vi "CRYControlCRY6181.vi"(0 "Command":string) -> (3 "Success?":bool, 4 "Margin":dbl, 6 "Table":string, 8 "Xdatapoints":dbl[](array[numeric]), 10 "Ydatapoints":dbl[](array[numeric]), 14 "Pass?":bool, 15 "Zdatapoints":dbl[](array[numeric]))   [LabVIEW 2013]
uses:
  CRYProject/CRYProject Editor Global.vi
  CRYMainGlobal.vi
  CRYWindow/SubVI/CRYMain Sub Window Global.vi
  CRYSystem/Task Sequence/CRYProject Run Control Global.vi
panel:
  # "run\nlot 121\nserial N1223\nexit\nopen I:\\__Test Sequence\\TSR THD.cry\ncurve Fundamental Harmonic \nnames"
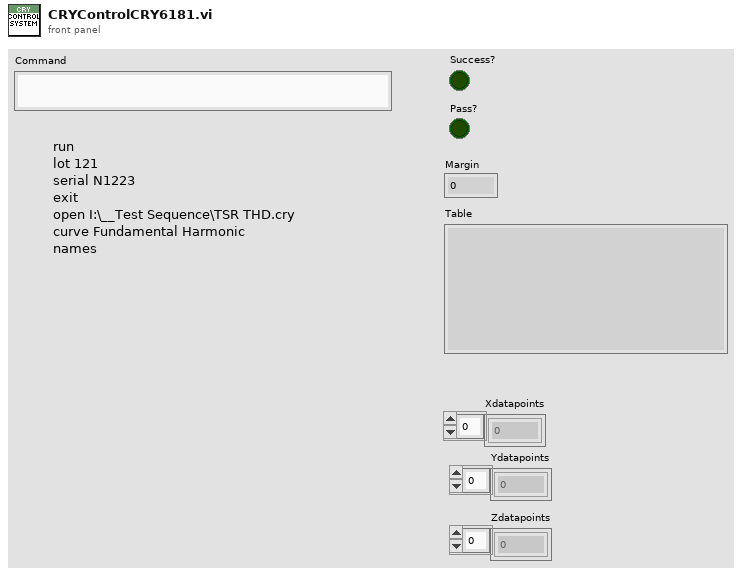
[diagram p1: front panel]
types:
  T1 = typedef "CRYData Cluster.ctl" = cluster{"Name":string, "Curve":cluster{"x":dbl, "y":dbl, "z":dbl}[], "X data":u16, "Y data":u16, "Z data":u16, "X axis":u16, "Y axis":u16, "Z axis":u16, "X unit":string, "Y unit":string, "Z unit":string, "X dB ref":dbl, "Y dB ref":dbl, "Z dB ref":dbl, "single val":bool, "protected":bool, "display X":bool, "display Y":bool, "display Z":bool, "Test Info":string, "Step No.":i32, "Plot Settings":cluster{"Color":u32, "Interpolation":u8, "Point Style":u8, "Line Style":u8, "Point Color":u32, "Line Width":u8, "Bar Plot Style":u8, "Fill To":i16}, "AutoProtect":bool}
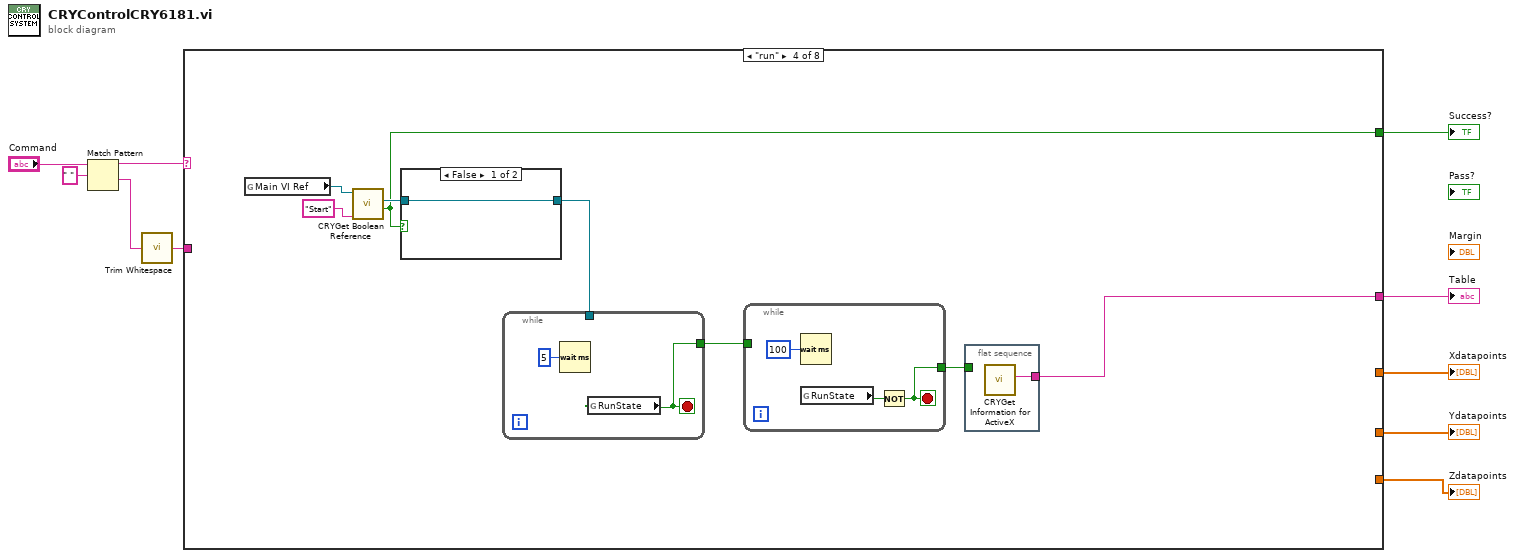
[diagram p0: block diagram]
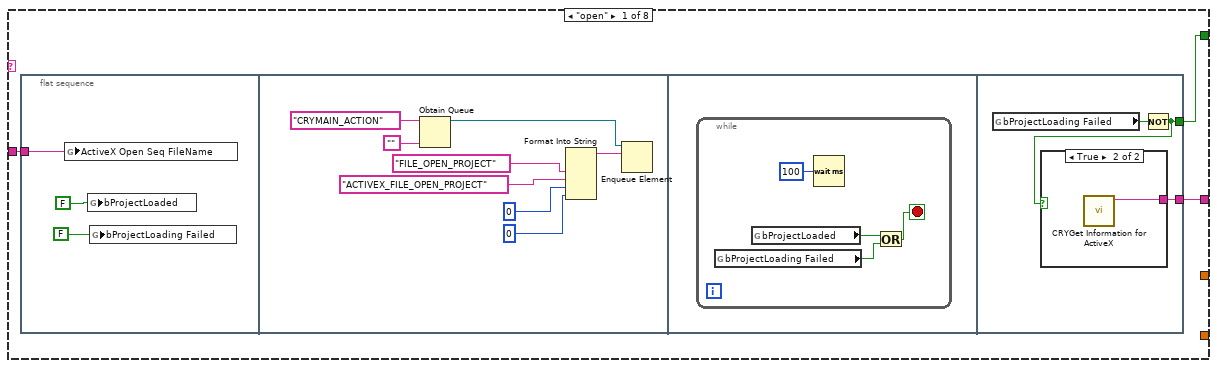
[diagram p2: hidden frame]
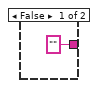
[diagram p3: hidden frame]
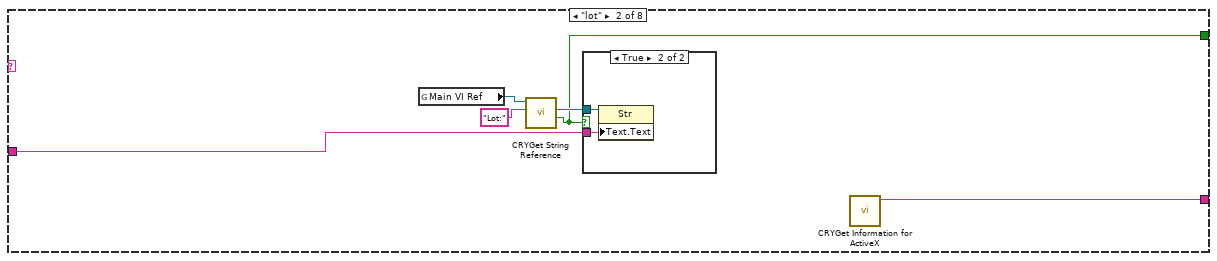
[diagram p4: hidden frame]
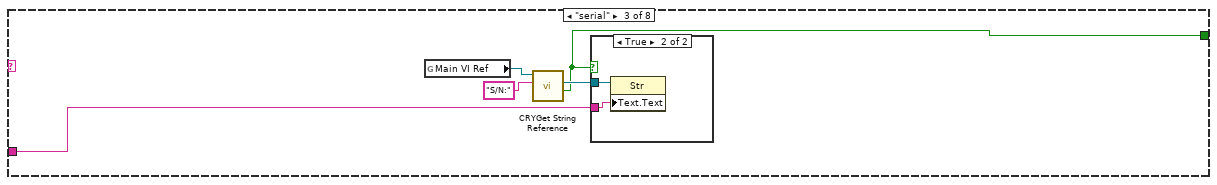
[diagram p6: hidden frame]
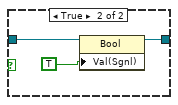
[diagram p8: hidden frame]
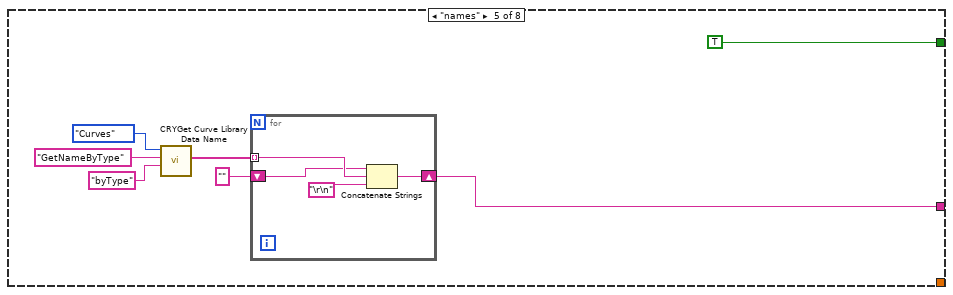
[diagram p9: hidden frame]
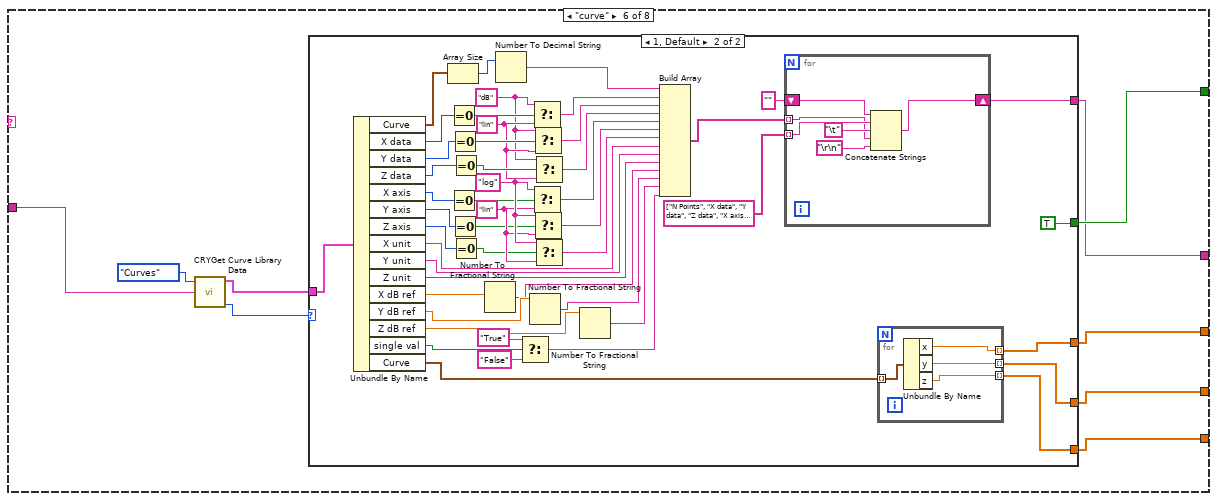
[diagram p10: hidden frame]
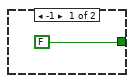
[diagram p11: hidden frame]
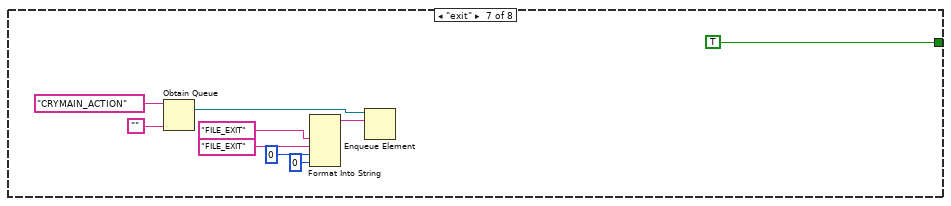
[diagram p12: hidden frame]
diagram:
  n1 = Match Pattern(string="Command", regular expression=" " ("search string/char (-)")) -> (before substring=w3:string, after substring=w2:string)  [unwired: 1 in, 2 out]
  n2 = call <vilib>:"Trim Whitespace.vi"("string"=w2) -> ("trimmed string"=w1:string)  [unwired: 1 in]
  n3 = case shown="\"run\"" w3 {
    tunnel: [w12 w34 _ w52 w68 w81 _ _] -> w10
    tunnel: [w11 w36 w43 w53 TRUE ("Boolean") w82 TRUE ("Boolean") _] -> w9
    tunnel: [_ _ _ _ _ w80 _ _] -> w8
    tunnel: [_ _ _ _ _ w79 _ _] -> w7
    tunnel: [_ _ _ _ _ w78 _ _] -> w6
    tunnel: w1 -> [w13 w35 w42 _ _ w85 _ _]
    frame "open" {
      n4 = flat-sequence {
        tunnel: w13 -> [w16]
        tunnel: [w31] -> w12
        tunnel: [w29] -> w11
        frame #0 {
          n5 = global write "CRYMainGlobal.vi" "ActiveX Open Seq FileName"(w16) -> ()
          n6 = global write "CRYProject Editor Global.vi" "bProjectLoaded"(FALSE (".not. x?")) -> ()
          n7 = global write "CRYProject Editor Global.vi" "bProjectLoading Failed"(FALSE ("bProjectLoaded Failed")) -> ()
        }
        frame #1 {
          n8 = Obtain Queue(name (unnamed)="CRYMAIN_ACTION" ("YAxisTitle"), element data type="" ("Action Type")) -> (queue out=w18:refnum<queue>)  [unwired: 3 in, 2 out]
          n9 = Format Into String("FILE_OPEN_PROJECT" ("input 1"), "ACTIVEX_FILE_OPEN_PROJECT" ("input 2"), 0 ("input 2"), 0 ("input 3")) -> (resulting string=w23:string)  [unwired: 3 in, 1 out]
          n10 = Enqueue Element(queue=w18, element=w23) -> ()  [unwired: 1 in, 4 out]
        }
        frame #2 {
          n11 = while {
            stop <- w25 stop-if-true
            n12 = global read "CRYProject Editor Global.vi" "bProjectLoading Failed"() -> (w26:bool)
            n13 = global read "CRYProject Editor Global.vi" "bProjectLoaded"() -> (w27:bool)
            n14 = Wait (ms)(milliseconds to wait=u32 100) -> ()  [unwired: 1 out]
            n15 = Or(x=w27, y=w26) -> (x .or. y?=w25:bool)
          }
        }
        frame #3 {
          n16 = global read "CRYProject Editor Global.vi" "bProjectLoading Failed"() -> (w30:bool)
          n17 = Not(x=w30) -> (.not. x?=w29:bool)
          n18 = case shown="True" w29 {
            tunnel: ["" ("Sequence Array Out") w33] -> w31
            frame False {
            }
            frame True {
              n19 = call "CRYGet Information for ActiveX.vi"() -> ("Sequence Array Out"=w33:string)  [unwired: 10 in, 1 out]
            }
          }
        }
      }
    }
    frame "lot" {
      n20 = global read "CRYMain Sub Window Global.vi" "Main VI Ref"() -> (w39:refnum<vi>)
      n21 = call "CRYGet String Reference.vi"("Label Name"="Lot:", "VI Refnum"=w39) -> ("Find?"=w36:bool, "String Ref Out"=w37:refnum<vi>)  [unwired: 7 in, 1 out]
      n22 = case shown="True" w36 {
        tunnel: w37 -> [_ w41]
        tunnel: w35 -> [_ w40]
        frame False {
        }
        frame True {
          n23 = property class="Str"(reference=w41, "Text.Text"=w40) -> ()  [unwired: 1 in, 2 out]
        }
      }
      n24 = call "CRYGet Information for ActiveX.vi"() -> ("Sequence Array Out"=w34:string)  [unwired: 10 in, 1 out]
    }
    frame "serial" {
      n25 = global read "CRYMain Sub Window Global.vi" "Main VI Ref"() -> (w46:refnum<vi>)
      n26 = call "CRYGet String Reference.vi"("Label Name"="S/N:", "VI Refnum"=w46) -> ("Find?"=w43:bool, "String Ref Out"=w44:refnum<vi>)  [unwired: 7 in, 1 out]
      n27 = case shown="True" w43 {
        tunnel: w44 -> [_ w48]
        tunnel: w42 -> [_ w47]
        frame False {
        }
        frame True {
          n28 = property class="Str"(reference=w48, "Text.Text"=w47) -> ()  [unwired: 1 in, 2 out]
        }
      }
    }
    frame "run" {
      n29 = global read "CRYMain Sub Window Global.vi" "Main VI Ref"() -> (w56:refnum<vi>)
      n30 = call "CRYGet Boolean Reference.vi"("Label Name"="Start", "VI Refnum"=w56) -> ("Exist?"=w53:bool, "Boolean Ref"=w54:refnum<vi>)  [unwired: 7 in, 1 out]
      n31 = case shown="False" w53 {
        tunnel: w54 -> [w63 w66]
        tunnel: [w63 w64] -> w50
        frame False {
        }
        frame True {
          n32 = property class="Bool"(reference=w66, "Val(Sgnl)"=TRUE ("Boolean")) -> (reference out=w64:refnum<vi>)  [unwired: 1 in, 1 out]
        }
      }
      n33 = while {
        tunnel: [w57] -> w49
        tunnel: w50 -> [_]
        stop <- w57 stop-if-true
        n34 = Wait (ms)(milliseconds to wait=u32 5) -> ()  [unwired: 1 out]
        n35 = global read "CRYProject Run Control Global.vi" "RunState"() -> (w57:bool)
      }
      n36 = while {
        tunnel: [w60] -> w51
        tunnel: w49 -> [_]
        stop <- w60 stop-if-true
        n37 = Wait (ms)(milliseconds to wait=u32 100) -> ()  [unwired: 1 out]
        n38 = global read "CRYProject Run Control Global.vi" "RunState"() -> (w62:bool)
        n39 = Not(x=w62) -> (.not. x?=w60:bool)
      }
      n40 = flat-sequence {
        tunnel: [w59] -> w52
        tunnel: w51 -> [_]
        frame #0 {
          n41 = call "CRYGet Information for ActiveX.vi"() -> ("Limit Array Out"=w59:string)  [unwired: 10 in, 1 out]
        }
      }
    }
    frame "names" {
      n42 = call "CRYGet Curve Library Data Name.vi"("sOption"="byType", "sAction"="GetNameByType", "Type"=enum16{"Curves", "Values", "Results", "WFM"}."Curves") -> ("sNames"=w72:string[])  [unwired: 5 in, 3 out]
      n43 = for {
        tunnel: w72 -> [w77] mode=indexing
        shift-right: [w74] -> w68
        shift-left: "" ("sOption") -> [w75]
        n44 = Concatenate Strings(w75, w77, "\r\n") -> (w74:string)
      }
    }
    frame "curve" {
      n45 = call "CRYGet Curve Library Data.vi"("Type"=enum16{"Curves", "Values", "Results", "WFM"}."Curves", "Data Name"=w85) -> ("Curve"=w84:T1, "index"=w83:i32)  [unwired: 3 out]
      n46 = case shown="1, Default" w83 {
        tunnel: w84 -> [_ w135]
        tunnel: [FALSE ("Boolean") TRUE ("Boolean")] -> w82
        tunnel: [_ w133] -> w80
        tunnel: [_ w132] -> w79
        tunnel: [_ w131] -> w78
        tunnel: [_ w88] -> w81
        frame -1 {
        }
        frame 1, Default {
          w119 = "lin"
          w120 = "log"
          w122 = "lin"
          w121 = "dB"
          n47 = Unbundle By Name(w135) -> ("Curve"=w130:cluster{"x":dbl, "y":dbl, "z":dbl}[], "X data"=w128:u16, "Y data"=w125:u16, "Z data"=w126:u16, "X axis"=w115:u16, "Y axis"=w114:u16, "Z axis"=w113:u16, "X unit"=w105:string, "Y unit"=w104:string, "Z unit"=w103:string, "X dB ref"=w102:dbl, "Y dB ref"=w101:dbl, "Z dB ref"=w100:dbl, "single val"=w98:bool, "Curve"=w99:cluster{"x":dbl, "y":dbl, "z":dbl}[])
          n48 = Array Size(array=w130) -> (size(s)=w129:i32)
          n49 = Equal To 0?(x=w128) -> (x = 0?=w127:bool)
          n50 = Equal To 0?(x=w115) -> (x = 0?=w116:bool)
          n51 = Equal To 0?(x=w125) -> (x = 0?=w124:bool)
          n52 = Equal To 0?(x=w114) -> (x = 0?=w117:bool)
          n53 = Equal To 0?(x=w126) -> (x = 0?=w123:bool)
          n54 = Equal To 0?(x=w113) -> (x = 0?=w118:bool)
          n55 = Number To Fractional String(number=w102) -> (F-format string=w95:string)  [unwired: 3 in]
          n56 = Number To Decimal String(number=w129) -> (decimal integer string=w112:string)  [unwired: 1 in]
          n57 = Select(t="True", s=w98, f="False") -> (s? t:f=w92:string)
          n58 = Number To Fractional String(number=w101) -> (F-format string=w94:string)  [unwired: 3 in]
          n59 = Select(t=w121, s=w127, f=w122) -> (s? t:f=w111:string)
          n60 = Select(t=w120, s=w116, f=w119) -> (s? t:f=w108:string)
          n61 = Select(t=w121, s=w124, f=w122) -> (s? t:f=w110:string)
          n62 = Select(t=w120, s=w117, f=w119) -> (s? t:f=w107:string)
          n63 = Select(t=w121, s=w123, f=w122) -> (s? t:f=w109:string)
          n64 = Select(t=w120, s=w118, f=w119) -> (s? t:f=w106:string)
          n65 = Number To Fractional String(number=w100) -> (F-format string=w93:string)  [unwired: 3 in]
          n66 = Build Array(w112, w111, w110, w109, w108, w107, w106, w105, w104, w103, w95, w94, w93, w92) -> (w90:string[])
          n67 = for {
            tunnel: string[] ["N Points", "X data", "Y data", "Z data", "X axis", "Y axis", "Z axis", "X unit", "Y unit", "Z unit", "X dB ref", "Y dB ref", "Z dB ref", "Sigle val?"] -> [w141] mode=indexing
            tunnel: w90 -> [w139] mode=indexing
            shift-right: [w138] -> w88
            shift-left: "" -> [w136]
            n68 = Concatenate Strings(w136, w141, "\t", w139, "\r\n") -> (w138:string)
          }
          n69 = for {
            tunnel: w99 -> [w145] mode=indexing
            tunnel: [w144] -> w133 mode=indexing
            tunnel: [w143] -> w132 mode=indexing
            tunnel: [w142] -> w131 mode=indexing
            n70 = Unbundle By Name(w145) -> ("x"=w144:dbl, "y"=w143:dbl, "z"=w142:dbl)
          }
        }
      }
    }
    frame "exit" {
      n71 = Obtain Queue(name (unnamed)="CRYMAIN_ACTION" ("YAxisTitle"), element data type="" ("Action Type")) -> (queue out=w147:refnum<queue>)  [unwired: 3 in, 2 out]
      n72 = Format Into String("FILE_EXIT" ("input 1"), "FILE_EXIT" ("input 1"), 0 ("input 2"), 0 ("input 3")) -> (resulting string=w153:string)  [unwired: 3 in, 1 out]
      n73 = Enqueue Element(queue=w147, element=w153) -> ()  [unwired: 1 in, 4 out]
    }
    frame Default {
    }
  }
  "Success?" <- w9
  "Table" <- w10
  "Xdatapoints" <- w8
  "Ydatapoints" <- w7
  "Zdatapoints" <- w6
